vi "AMPM Fetch.vi"(0 "RFmx Handle In":refnum<k21>, 1 "Selector String":string, 11 "error in (no error)":errorcluster) -> (4 "RFmx Handle Out":refnum<k21>, 6 "AMPM Results":T1 {"AM to PM Residual (deg)" format="%.2f"; "AM to AM Residual (dB)" format="%.2f"; "Mean RMS EVM (%)" format="%.2f"; "1 dB Compression Point (dBm)" format="%.2f"; "Mean Linear Gain (dB)" format="%.2f"}, 15 "error out":errorcluster)   [LabVIEW 2016, in "RFmxSpecAn.lvlib"]
uses:
  RFmxSpecAn.lvlib
  Typedefs/AMPM Results.ctl
  <vilib>/RFmx/SpecAn/mx/RFmxSpecAn.llb/RFmxSpecAn AMPM Fetch DUT Characteristics.vi
  <vilib>/RFmx/SpecAn/mx/RFmxSpecAn.llb/RFmxSpecAn AMPM Fetch Curve Fit Residual.vi
  <vilib>/RFmx/SpecAn/mx/RFmxSpecAn.llb/RFmxSpecAn AMPM Fetch AM to AM Trace.vi
  <vilib>/RFmx/SpecAn/mx/RFmxSpecAn.llb/RFmxSpecAn AMPM Fetch AM to PM Trace.vi
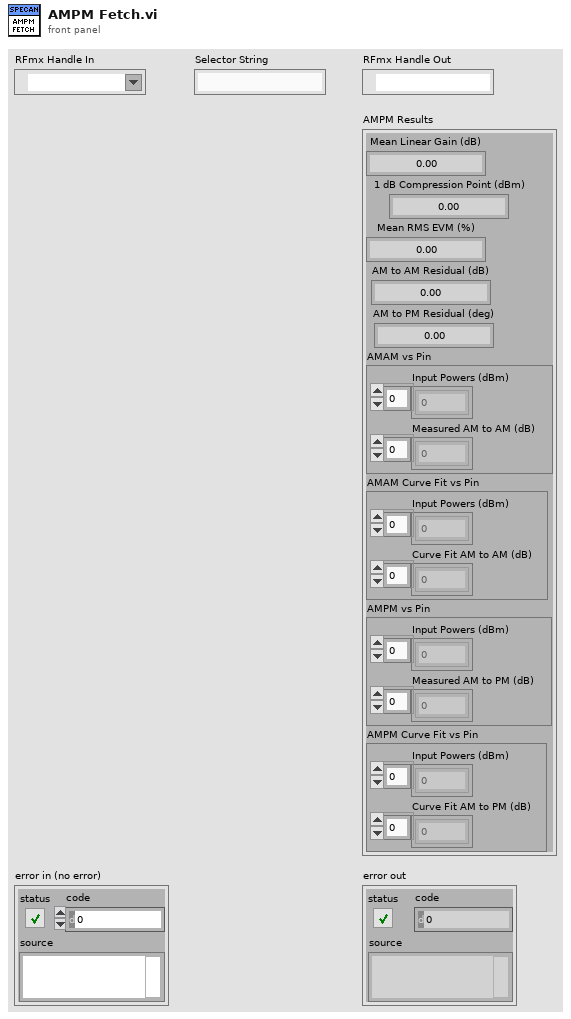
[diagram p1: front panel]
types:
  T1 = typedef "RFmxSpecAn.lvlib/AMPM Results.ctl" = cluster{"Mean Linear Gain (dB)":dbl, "1 dB Compression Point (dBm)":dbl, "Mean RMS EVM (%)":dbl, "AM to AM Residual (dB)":dbl, "AM to PM Residual (deg)":dbl, "AMAM vs Pin":cluster{"Input Powers (dBm)":sgl[], "Measured AM to AM (dB)":sgl[]}, "AMAM Curve Fit vs Pin":cluster{"Input Powers (dBm)":sgl[], "Curve Fit AM to AM (dB)":sgl[]}, "AMPM vs Pin":cluster{"Input Powers (dBm)":sgl[], "Measured AM to PM (dB)":sgl[]}, "AMPM Curve Fit vs Pin":cluster{"Input Powers (dBm)":sgl[], "Curve Fit AM to PM (dB)":sgl[]}}
  T2 = cluster{"Reference Powers (dBm)":sgl[], "Measured AM to AM (dB)":sgl[]}
  T3 = cluster{"Reference Powers (dBm)":sgl[], "Curve Fit AM to AM (dB)":sgl[]}
  T4 = cluster{"Reference Powers (dBm)":sgl[], "Measured AM to PM (deg)":sgl[]}
  T5 = cluster{"Reference Powers (dBm)":sgl[], "Curve Fit AM to PM (deg)":sgl[]}
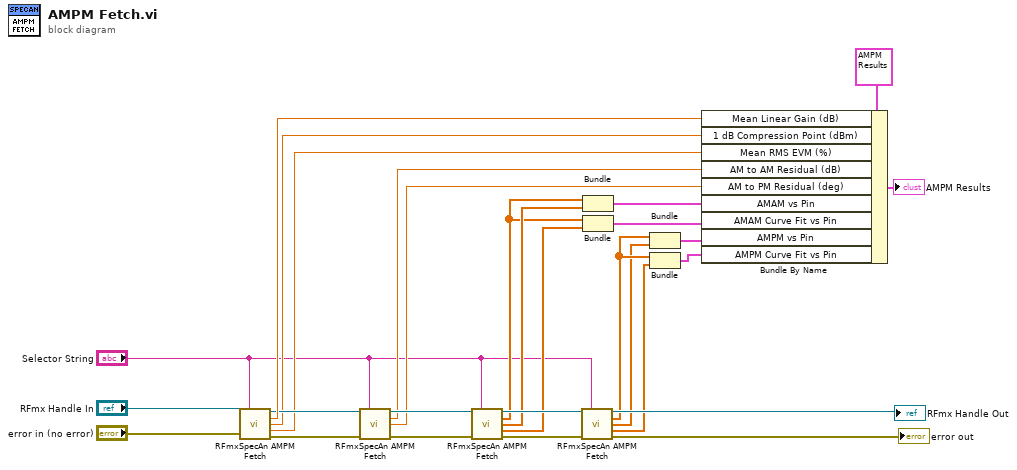
[diagram p0: block diagram]
diagram:
  n1 = call-poly <vilib>:"RFmxSpecAn AMPM Fetch.vi"("Instrument Handle In"="RFmx Handle In", "Selector String"="Selector String", "error in (no error)"="error in (no error)") -> ("Instrument Handle Out"=w23:refnum<k21>, "Mean Linear Gain (dB)"=w26:dbl, "1 dB Compression Point (dBm)"=w16:dbl, "Mean RMS EVM (%)"=w15:dbl, "error out"=w28:errorcluster)  [unwired: 8 in]
  n2 = call-poly <vilib>:"RFmxSpecAn AMPM Fetch.vi"("Instrument Handle In"=w23, "Selector String"="Selector String", "error in (no error)"=w28) -> ("Instrument Handle Out"=w21:refnum<k21>, "AM to AM Residual (dB)"=w14:dbl, "AM to PM Residual (deg)"=w13:dbl, "error out"=w24:errorcluster)  [unwired: 9 in]
  n3 = call-poly <vilib>:"RFmxSpecAn AMPM Fetch.vi"("Instrument Handle In"=w21, "Selector String"="Selector String", "error in (no error)"=w24) -> ("Instrument Handle Out"=w19:refnum<k21>, "Reference Powers (dBm)"=w10:sgl[], "Measured AM to AM (dB)"=w17:sgl[], "Curve Fit AM to AM (dB)"=w11:sgl[], "error out"=w22:errorcluster)  [unwired: 8 in]
  n4 = call-poly <vilib>:"RFmxSpecAn AMPM Fetch.vi"("Instrument Handle In"=w19, "Selector String"="Selector String", "error in (no error)"=w22) -> ("Instrument Handle Out"=→"RFmx Handle Out":refnum<k21>, "Reference Powers (dBm)"=w6:sgl[], "Measured AM to PM (deg)"=w5:sgl[], "Curve Fit AM to PM (deg)"=w4:sgl[], "error out"=→"error out":errorcluster)  [unwired: 8 in]
  n5 = Bundle("Reference Powers (dBm)"=w10, "Measured AM to AM (dB)"=w17) -> (w12:T2)  [unwired: 1 in]
  n6 = Bundle("Reference Powers (dBm)"=w10, "Curve Fit AM to AM (dB)"=w11) -> (w9:T3)  [unwired: 1 in]
  n7 = Bundle("Reference Powers (dBm)"=w6, "Measured AM to PM (deg)"=w5) -> (w8:T4)  [unwired: 1 in]
  n8 = Bundle("Reference Powers (dBm)"=w6, "Curve Fit AM to PM (deg)"=w4) -> (w7:T5)  [unwired: 1 in]
  n9 = Bundle By Name(cluster=T1 {"Mean Linear Gain (dB)"=0.0, "1 dB Compression Point (dBm)"=0.0, "Mean RMS EVM (%)"=0.0, "AM to AM Residual (dB)"=0.0, "AM to PM Residual (deg)"=0.0, "AMAM vs Pin"={"Input Powers (dBm)"=[], "Measured AM to AM (dB)"=[]}, "AMAM Curve Fit vs Pin"={"Input Powers (dBm)"=[], "Curve Fit AM to AM (dB)"=[]}, "AMPM vs Pin"={"Input Powers (dBm)"=[], "Measured AM to PM (dB)"=[]}, "AMPM Curve Fit vs Pin"={"Input Powers (dBm)"=[], "Curve Fit AM to PM (dB)"=[]}} ("AMPM Results"), "Mean Linear Gain (dB)"=w26, "1 dB Compression Point (dBm)"=w16, "Mean RMS EVM (%)"=w15, "AM to AM Residual (dB)"=w14, "AM to PM Residual (deg)"=w13, "AMAM vs Pin"=w12, "AMAM Curve Fit vs Pin"=w9, "AMPM vs Pin"=w8, "AMPM Curve Fit vs Pin"=w7) -> (→"AMPM Results":T1)
